vi "Packet Read.vi"(11 "Packets":string) -> (0 "Digital IO":bool[](array[boolean]), 3 "Analog Channels":cluster{u16, u16, u16, u16, u16, u16}, 4 "Sequential Number":u8, 5 "CRC Error":bool)   [LabVIEW 2015]
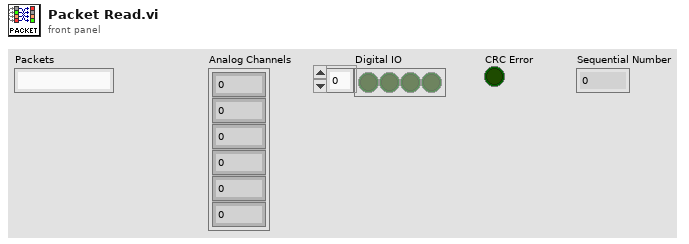
[diagram p1: front panel]
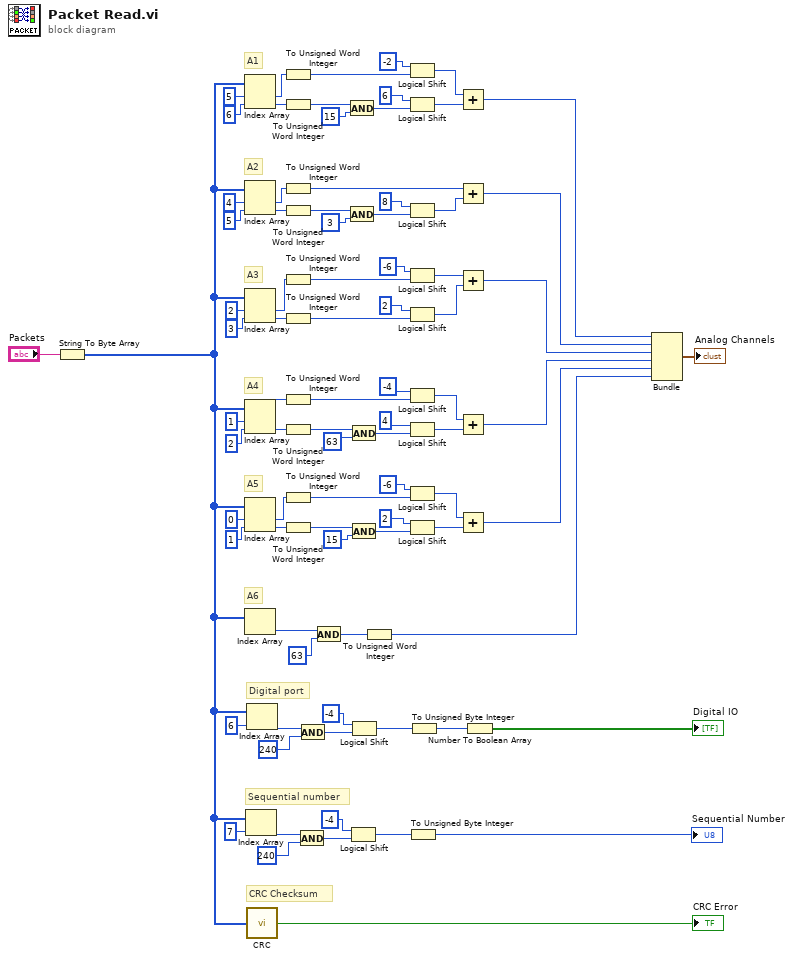
[diagram p0: block diagram]
diagram:
  # "CRC Checksum"
  # "Digital port"
  # "Sequential number"
  # "A6"
  # "A5"
  # "A4"
  # "A3"
  # "A2"
  # "A1"
  n1 = String To Byte Array(string="Packets") -> (unsigned byte array=w2:u8[])
  n2 = Index Array(array=w2, index #1=5 ("index"), index #2=6 ("index")) -> (element #1=w79:u8, element #2=w81:u8)
  n3 = Index Array(array=w2, index #1=4 ("index"), index #2=5 ("index")) -> (element #1=w69:u8, element #2=w71:u8)
  n4 = Index Array(array=w2, index #1=2 ("index"), index #2=3 ("index")) -> (element #1=w54:u8, element #2=w61:u8)
  n5 = Index Array(array=w2, index #1=1 ("index"), index #2=2 ("index")) -> (element #1=w48:u8, element #2=w51:u8)
  n6 = Index Array(array=w2, index #1=0 ("index"), index #2=1 ("index")) -> (element #1=w36:u8, element #2=w39:u8)
  n7 = Index Array(array=w2) -> (element=w27:u8)  [unwired: 1 in]
  n8 = Index Array(array=w2, index=7) -> (element=w18:u8)
  n9 = Index Array(array=w2, index=6) -> (element=w11:u8)
  n10 = call "CRC.vi"("Packet byte array"=w2) -> ("CRC Error"=→"CRC Error":bool)
  n11 = To Unsigned Word Integer(number=w79) -> (unsigned 16bit integer=w78:u16)
  n12 = To Unsigned Word Integer(number=w81) -> (unsigned 16bit integer=w80:u16)
  n13 = To Unsigned Word Integer(number=w69) -> (unsigned 16bit integer=w67:u16)
  n14 = To Unsigned Word Integer(number=w71) -> (unsigned 16bit integer=w66:u16)
  n15 = To Unsigned Word Integer(number=w54) -> (unsigned 16bit integer=w57:u16)
  n16 = To Unsigned Word Integer(number=w61) -> (unsigned 16bit integer=w60:u16)
  n17 = To Unsigned Word Integer(number=w48) -> (unsigned 16bit integer=w47:u16)
  n18 = To Unsigned Word Integer(number=w51) -> (unsigned 16bit integer=w44:u16)
  n19 = To Unsigned Word Integer(number=w36) -> (unsigned 16bit integer=w35:u16)
  n20 = To Unsigned Word Integer(number=w39) -> (unsigned 16bit integer=w32:u16)
  n21 = And(x=w18, y=u8 240) -> (x .and. y?=w16:u8)
  n22 = And(x=w11, y=u8 240) -> (x .and. y?=w9:u8)
  n23 = And(x=w27, y=u8 63) -> (x .and. y?=w25:u8)
  n24 = And(x=w80, y=u16 15) -> (x .and. y?=w76:u16)
  n25 = And(x=w66, y=u16 3) -> (x .and. y?=w64:u16)
  n26 = Logical Shift(y=i16 -4, x=w16) -> (x << y=w15:u8)
  n27 = And(x=w44, y=u16 63) -> (x .and. y?=w43:u16)
  n28 = And(x=w32, y=u16 15) -> (x .and. y?=w31:u16)
  n29 = Logical Shift(y=i16 -4, x=w9) -> (x << y=w8:u8)
  n30 = To Unsigned Word Integer(number=w25) -> (unsigned 16bit integer=w19:u16)
  n31 = Logical Shift(y=i16 -2, x=w78) -> (x << y=w75:u16)
  n32 = Logical Shift(y=u16 6, x=w76) -> (x << y=w74:u16)
  n33 = Logical Shift(y=u16 8, x=w64) -> (x << y=w68:u16)
  n34 = Logical Shift(y=i16 -6, x=w57) -> (x << y=w55:u16)
  n35 = Logical Shift(y=u16 2, x=w60) -> (x << y=w58:u16)
  n36 = Logical Shift(y=i16 -4, x=w47) -> (x << y=w45:u16)
  n37 = Logical Shift(y=u16 4, x=w43) -> (x << y=w49:u16)
  n38 = Logical Shift(y=i16 -6, x=w35) -> (x << y=w33:u16)
  n39 = Logical Shift(y=u16 2, x=w31) -> (x << y=w37:u16)
  n40 = To Unsigned Byte Integer(number=w15) -> (unsigned 8bit integer=→"Sequential Number":u8)
  n41 = To Unsigned Byte Integer(number=w8) -> (unsigned 8bit integer=w5:u8)
  n42 = Add(x=w75, y=w74) -> (x+y=w24:u16)
  n43 = Add(x=w67, y=w68) -> (x+y=w23:u16)
  n44 = Add(x=w55, y=w58) -> (x+y=w22:u16)
  n45 = Add(x=w45, y=w49) -> (x+y=w21:u16)
  n46 = Add(x=w33, y=w37) -> (x+y=w20:u16)
  n47 = Number To Boolean Array(number=w5) -> (Boolean array=→"Digital IO":bool[])
  n48 = Bundle(w24, w23, w22, w21, w20, w19) -> (→"Analog Channels":cluster{u16, u16, u16, u16, u16, u16})  [unwired: 1 in]
